vi "Endurance PWM Initialization.vi"() -> (3 "Array":u8[](array[numeric]))   [LabVIEW 2011]
panel:
  # "This SubVI initalializes an array with 9 entries - the first (entry 0) should always be 0.\nThe next 8 channels correspond to an output port on Endurance and should give the\nPMW's a value between 0 and 255"
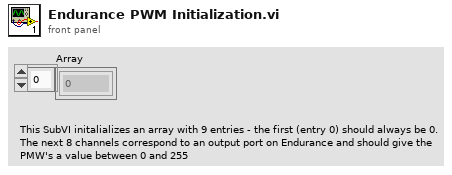
[diagram p1: front panel]
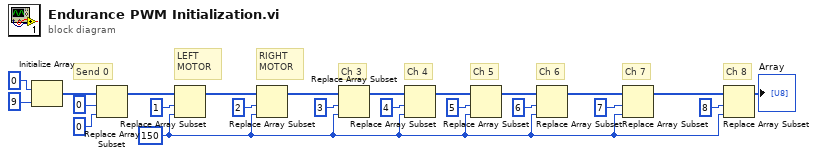
[diagram p0: block diagram]
diagram:
  w22 = u8 150 ("new element/subarray")
  # "RIGHT\nMOTOR"
  # "LEFT\nMOTOR"
  # "Send 0"
  # "Ch 8"
  # "Ch 7"
  # "Ch 6"
  # "Ch 5"
  # "Ch 4"
  # "Ch 3"
  n1 = Initialize Array(u8 0 ("element"), 9 ("dimension size")) -> (w20:u8[])
  n2 = Replace Array Subset(array=w20, new element=u8 0 ("new element/subarray"), index=0) -> (w16:u8[])
  n3 = Replace Array Subset(array=w16, new element=w22, index=1) -> (w17:u8[])
  n4 = Replace Array Subset(array=w17, new element=w22, index=2) -> (w21:u8[])
  n5 = Replace Array Subset(array=w21, new element=w22, index=3) -> (w12:u8[])
  n6 = Replace Array Subset(array=w12, new element=w22, index=4) -> (w3:u8[])
  n7 = Replace Array Subset(array=w3, new element=w22, index=5) -> (w2:u8[])
  n8 = Replace Array Subset(array=w2, new element=w22, index=6) -> (w9:u8[])
  n9 = Replace Array Subset(array=w9, new element=w22, index=7) -> (w7:u8[])
  n10 = Replace Array Subset(array=w7, new element=w22, index=8) -> (→"Array":u8[])
